vi "GetInitialDataMVP15.vi"(8 "error In":errorcluster, 10 "Adress":u16=1 max=999 step=1, 11 "VISA session":refnum<visa-resource-name>) -> (0 "error out":errorcluster, 2 "Map":map{T1, variant}(c390), 3 "VISA session Out":refnum<visa-resource-name>)   [LabVIEW 2019]
uses:
  PfeifferMVP15Cmds.ctl
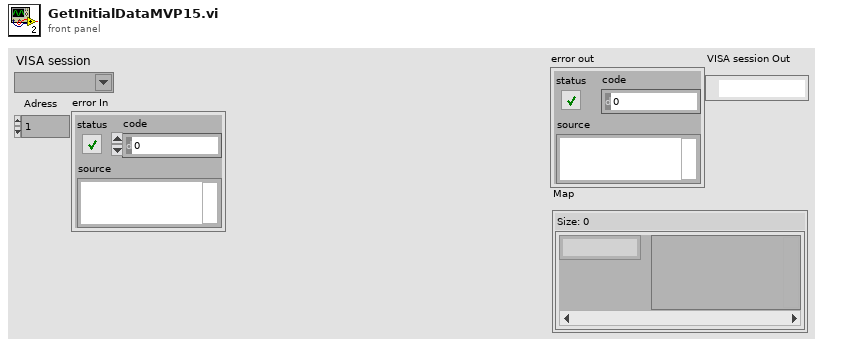
[diagram p1: front panel]
types:
  T1 = typedef "PfeifferMVP15Cmds.ctl" = enum16{"Standby", "Run", "AckError", "ErrorCode", "ActualSpdHz", "DrvCurrent", "OpHrsPump", "FwVersion", "DrvVoltage", "NominalSpdHz", "DrvPower", "ElecName", "HWVersion", "ActualSpdRPM", "NominalSpdRPM", "TempPump"}
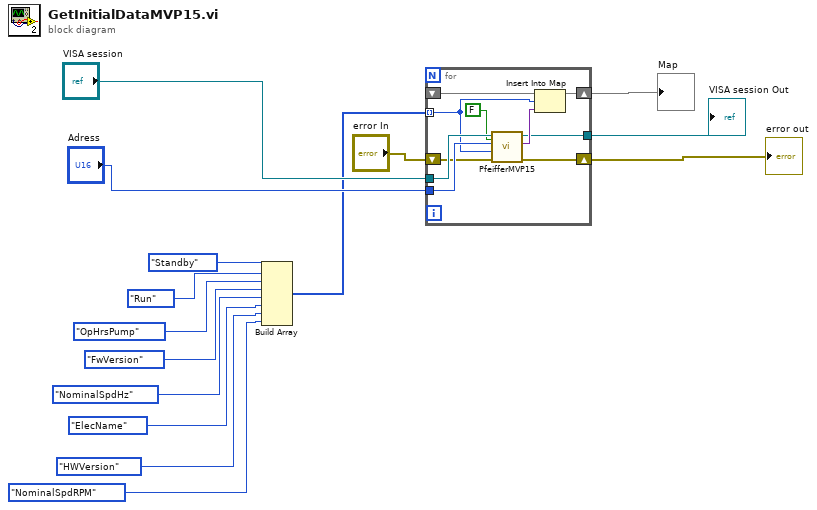
[diagram p0: block diagram]
diagram:
  n1 = Build Array(PfeifferMVP15Cmds."Standby" ("Cmd"), PfeifferMVP15Cmds."Run" ("Cmd"), PfeifferMVP15Cmds."OpHrsPump" ("Cmd"), PfeifferMVP15Cmds."FwVersion" ("Cmd"), PfeifferMVP15Cmds."NominalSpdHz" ("Cmd"), PfeifferMVP15Cmds."ElecName" ("Cmd"), PfeifferMVP15Cmds."HWVersion" ("Cmd"), PfeifferMVP15Cmds."NominalSpdRPM" ("Cmd")) -> (w5:T1[])
  n2 = for {
    tunnel: "VISA session" -> [w25]
    tunnel: "Adress" -> [w24]
    tunnel: w5 -> [w22] mode=indexing
    shift-right: [w20] -> w3
    shift-left: _ -> [w19]
    shift-right: [w18] -> w4
    shift-left: "error In" -> [w17]
    tunnel: [w16] -> w1
    n3 = call "PfeifferMVP15.vi"("Write?"=FALSE, "error in"=w17, "Cmd"=w22, "Adress"=w24, "VISA session"=w25) -> ("error out"=w18:errorcluster, "Result"=w21:variant, "VISA session Out"=w16:refnum<visa-resource-name>)  [unwired: 4 in]
    n4 = Insert Into Map(map in=w19, key=w22, value=w21) -> (map out=w20:map{T1, variant})  [unwired: 2 out]
  }
  "error out" <- w4
  "Map" <- w3
  "VISA session Out" <- w1
